vi "hmi_sistema_de_deteccion_de_fugas.vi"() -> ()   [LabVIEW 2017]
uses:
  Control 6.ctl
  <vilib>/Utility/miscctls.llb/LVBoundsTypeDef.ctl
  <vilib>/Instr/_visa.llb/VISA Configure Serial Port (Instr).vi
  <vilib>/MakerHub/LINX/LMH-LINX.lvlib
panel:
  in  "Tab Control":enum32{"HMI", "Monitorizacion de flujo"}(tab)
  out "Boolean 2":bool
  out "FUGA 1":bool
  out "FUGA 2":bool
  out "Boolean":bool
  in  "stop 2":bool
  in  "BOMBA ON/OFF":bool
  out "FT1":bool(c317)
  out "TANQUE\n FLUIDO:AGUA":dbl(slide) scale=0.0..100.0
  in  "valvula 1":bool
  in  "valvula 2":bool
  out "TEE 02":bool
  out "TUBERIA 1IN TRAMO 02":bool(c317)
  out "TEE1":bool
  out "Multi-Segment Pipe 2":T1
  out "Multi-Segment Pipe 3":bool(c317)
  out "BOMBA 1/2 HP":bool
  out "codo90":bool
  out "Multi-Segment Pipe 4":bool(c317)
  out "FT2":bool(c317)
  out "FT 1":dbl caption="L/min"
  out "FT 2":dbl caption="L/min"
  out "67.5°":bool
  out "45°":bool
  out "22.5°":bool
  out "90°":bool
  out "SENSOR FLUJO":bool
  out "67.5° 3":bool
  out "45° 3":bool
  out "22.5° 3":bool
  out "90° 3":bool
  out "SENSOR FLUJO 3":bool
  in  "Tiempo de Muestreo":string(combo)
  in  "Jump Button 4":bool
  in  "Guardar  a Excel":bool
  in  "Rango de grafica":i16(knob) scale=0.0..100.0
  out "Flujo de entrada y salida":cluster{dbl[], dbl[]}[](graph)
  out "Tiempo de Muestreo":dbl caption="s"
  in  "Jump Button 3":bool
  in  "stop":bool
  out "Freq2":dbl
  out "Freq1":dbl
  out "Cluster":T2
  in  "Puerto":refnum<visa-resource-name>="COM3"
  in  "BaudRate":i32(ring)=10 items=["9600"=9600, "19200"=19200, "38400"=38400, "57600"=57600, "74880"=74880, "115200"=115200]
  # "PVC  1\" FLUJO: AGUA"
  # "PVC  1/2\" FLUJO: AGUA"
  # "FUGA 1"
  # "2.5 m"
  # "PVC  1/2\" FLUJO: AGUA"
  # "FUGA 2"
  # "PVC  1\" FLUJO: AGUA"
  # "6 m"
  # "MONITOREO DE SENSORES DE FLUJO YF-S201"
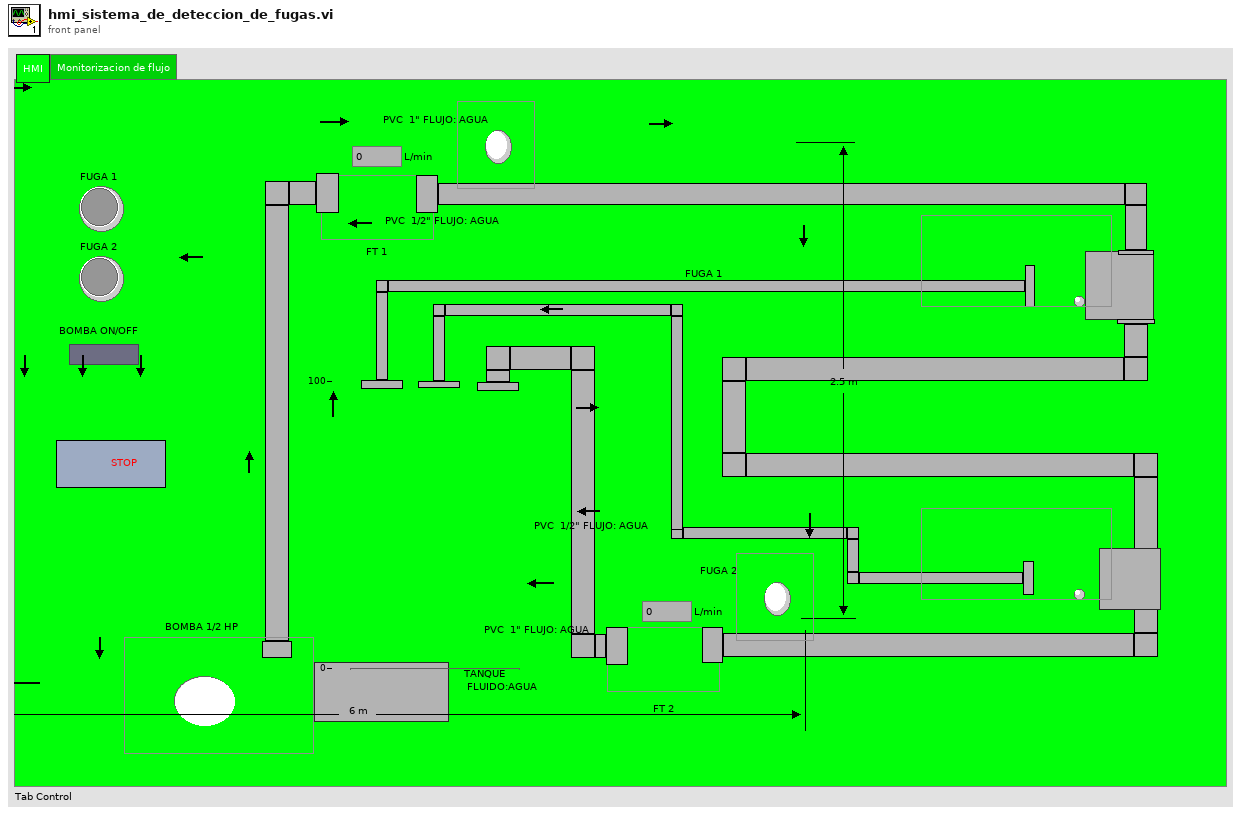
[diagram p1: front panel]
types:
  T1 = typedef "Control 6.ctl" = bool
  T2 = cluster{"FLUJO DE ENTRADA":dbl, "FLUJO DE SALIDA":dbl, "VOLUMEN 1 (L) ":dbl, "VOLUMEN 2 (L) ":dbl}
  T3 = typedef "LVBoundsTypeDef.ctl" = cluster{"Width":u32, "Height":u32}
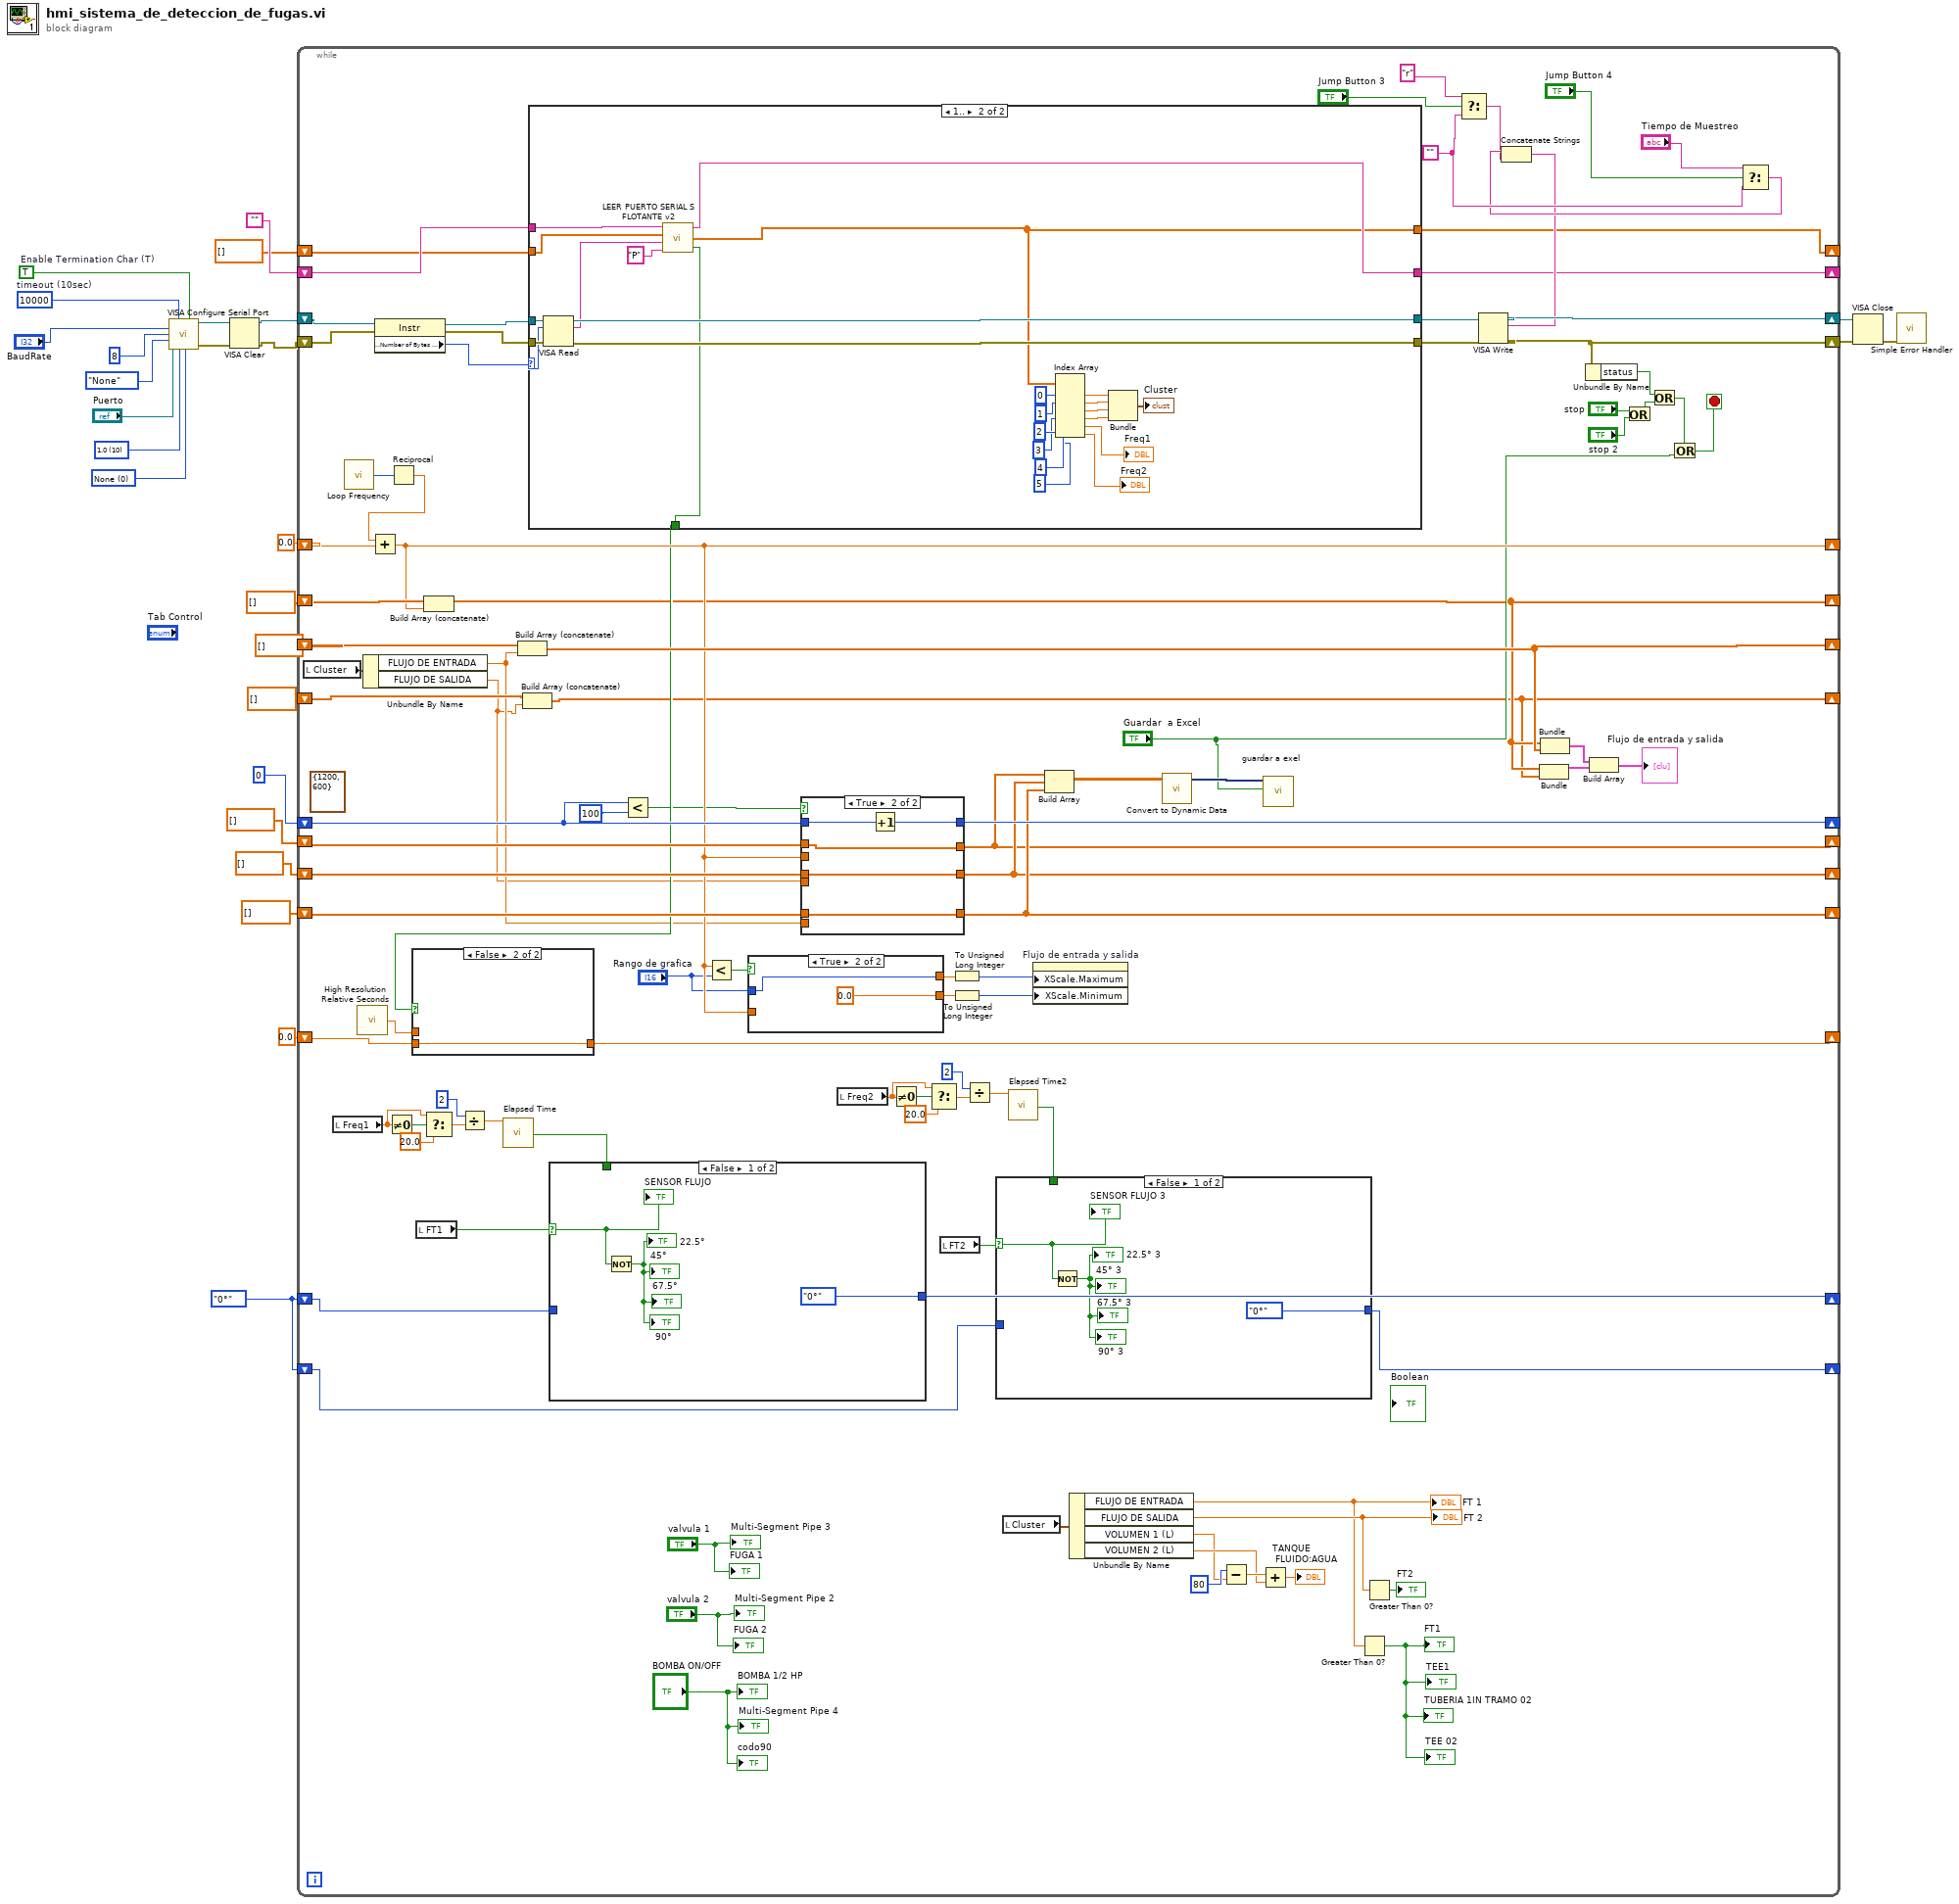
[diagram p0: block diagram]
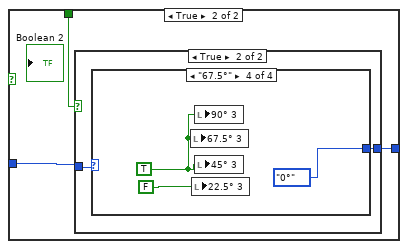
[diagram p2: hidden frame]
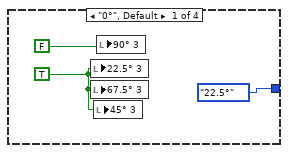
[diagram p4: hidden frame]
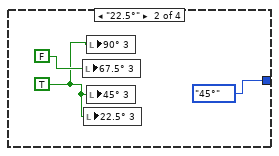
[diagram p5: hidden frame]
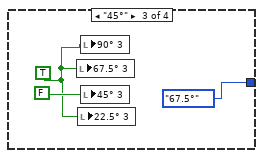
[diagram p6: hidden frame]
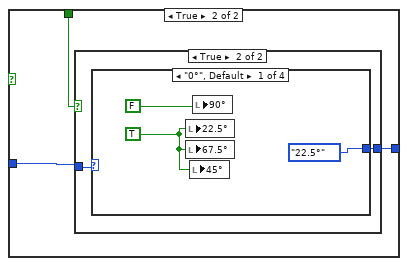
[diagram p7: hidden frame]
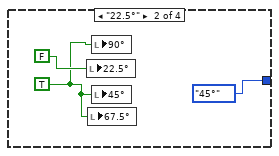
[diagram p9: hidden frame]
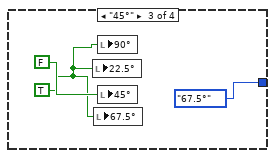
[diagram p10: hidden frame]
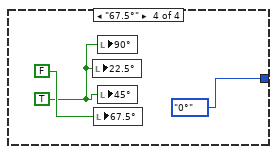
[diagram p11: hidden frame]
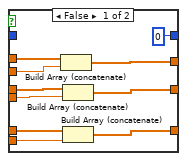
[diagram p12: hidden frame]
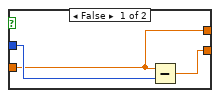
[diagram p13: hidden frame]
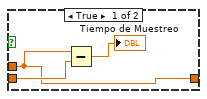
[diagram p14: hidden frame]
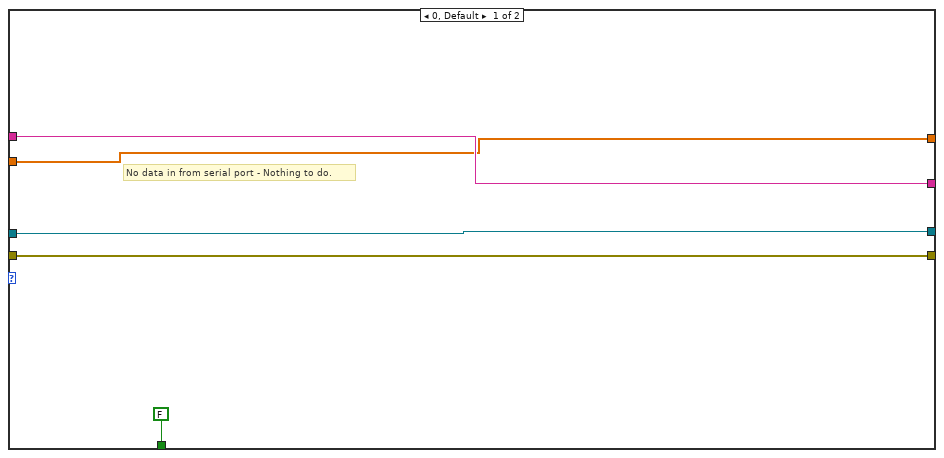
[diagram p15: hidden frame]
diagram:
  w3 = enum16{"0°", "22.5°", "45°", "67.5°"}."0°"
  w18 = u16 10 items=["1.0"=10, "1.5"=15, "2.0"=20] ("stop bits (10: 1 bit)")
  w19 = u16 0 items=["None", "XON/XOFF", "RTS/CTS", "XON/XOFF & RTS/CTS", "DTR/DSR", "XON/XOFF & DTR/DSR"] ("flow control (0:none)")
  w24 = TRUE  # Enable Termination Char (T)
  w25 = u32 10000  # timeout (10sec)
  (unwired) T3 {"Width"=1200, "Height"=600} ("Tab Control Pane Dimension")
  n1 = call-poly "VISA Configure Serial Port"("VISA resource name"="Puerto", "timeout (10sec)"=w25, "Enable Termination\nChar (T)"=w24, "baud rate (9600)"="BaudRate", "data bits (8)"=u16 8 ("Data bits (8)"), "parity (0:none)"=enum16{"None", "Odd", "Even", "Mark", "Space"}."None" ("Parity (0:none)"), "stop bits (10: 1 bit)"=w18, "flow control (0:none)"=w19) -> ("VISA resource name out"=w22:refnum<visa-resource-name>, "error out"=w23:errorcluster)  [unwired: 6 in]
  n2 = VISA Clear(VISA resource name=w22, error in (no error)=w23) -> (VISA resource name out=w21:refnum<visa-resource-name>, error out=w6:errorcluster)
  n3 = while {
    shift-right: [w72] -> _
    shift-left: dbl[] [] -> [w116]
    shift-right: [w93] -> _
    shift-left: 0.0 -> [w117]
    shift-right: [w104] -> _
    shift-left: dbl[] [] -> [w114]
    shift-right: [w71] -> _
    shift-left: dbl[] [] -> [w115]
    shift-right: [w112] -> _
    shift-left: 0.0 ("relative seconds") -> [w113]
    shift-right: [w99] -> _
    shift-left: 0 -> [w100]
    shift-right: [w94] -> _
    shift-left: dbl[] [] -> [w97]
    shift-right: [w95] -> _
    shift-left: dbl[] [] -> [w96]
    shift-right: [w92] -> _
    shift-left: dbl[] [] -> [w98]
    shift-right: [w119] -> w27
    shift-left: w6 -> [w87]
    shift-right: [w86] -> w5
    shift-left: w21 -> [w124]
    shift-right: [w57] -> _
    shift-left: w3 -> [w56]
    shift-right: [w37] -> _
    shift-left: w3 -> [w46]
    shift-right: [w30] -> _
    shift-left: "" -> [w31]
    shift-right: [w28] -> _
    shift-left: dbl[] [] -> [w29]
    stop <- w103 stop-if-true
    w85 = ""
    n4 = local read "Cluster"() -> (w70:T2)
    n5 = local read "Freq1"() -> (w54:dbl)
    n6 = call <vilib>:"Loop Frequency.vi"() -> ("Loop Rate (Hz)"=w107:u32)
    n7 = call <vilib>:"High Resolution Relative Seconds.vi"() -> ("relative seconds"=w108:dbl)
    n8 = Unbundle By Name(w70) -> ("FLUJO DE ENTRADA"=w69:dbl, "FLUJO DE SALIDA"=w68:dbl)
    n9 = property class="Instr"(reference=w124, error in=w87) -> (reference out=w126:refnum<visa-resource-name>, error out=w125:errorcluster, "Serial Settings:Number of Bytes at Serial Port"=w123:u32)
    n10 = Not Equal To 0?(x=w54) -> (x != 0?=w55:bool)
    n11 = Reciprocal(x=w107) -> (1/x=w111:dbl)
    n12 = Add(x=w111, y=w117) -> (x+y=w93:dbl)
    n13 = local read "FT1"() -> (w58:bool)
    n14 = Build Array (concatenate)(w116, w93) -> (w72:dbl[])
    n15 = Select(t=w54, s=w55, f=20.0) -> (s? t:f=w52:dbl)
    n16 = Divide(x=i8 2, y=w52) -> (x/y=w51:dbl)
    n17 = call "Elapsed Time"("Time Target (s)"=w51) -> ("Time has Elapsed"=w49:bool)  [unwired: 11 in, 7 out]
    n18 = Build Array (concatenate)(w114, w69) -> (w104:dbl[])
    n19 = Build Array (concatenate)(w115, w68) -> (w71:dbl[])
    n20 = case shown="1.." w123 {
      selector: w123 -> [_ w218]
      tunnel: [w196 w222] -> w120
      tunnel: [w197 w221] -> w121
      tunnel: w126 -> [w197 w220]
      tunnel: w125 -> [w196 w219]
      tunnel: [FALSE w203] -> w88
      tunnel: w31 -> [w194 w201]
      tunnel: [w194 w200] -> w30
      tunnel: w29 -> [w193 w199]
      tunnel: [w193 w198] -> w28
      frame 0, Default {
        # "No data in from serial port - Nothing to do."
      }
      frame 1.. {
        n21 = VISA Read(VISA resource name=w220, byte count=w218, error in (no error)=w219) -> (VISA resource name out=w221:refnum<visa-resource-name>, read buffer=w202:string, error out=w222:errorcluster)  [unwired: 1 out]
        n22 = call <userlib>:"LEER PUERTO SERIAL S FLOTANTE v2.vi"("caracter terminador"="P" ("regular expression"), "read buffer"=w202, "buffer de datos"=w199, "buffer in"=w201) -> ("indicador de llegada de datos"=w203:bool, "salida datos numericos"=w198:dbl[], "buffer out"=w200:string)
        n23 = Index Array(array=w198, index #1=0 ("index"), index #2=1 ("index"), index #3=2 ("index"), index #4=3 ("index"), index #5=4 ("index"), index #6=5 ("index")) -> (element #1=w216:dbl, element #2=w215:dbl, element #3=w213:dbl, element #4=w214:dbl, element #5=→"Freq1":dbl, element #6=→"Freq2":dbl)
        n24 = Bundle(w216, w215, w213, w214) -> (→"Cluster":cluster{dbl, dbl, dbl, dbl})  [unwired: 1 in]
      }
    }
    n25 = case shown="False" w88 {
      tunnel: w113 -> [w191 w192]
      tunnel: w108 -> [w189 _]
      tunnel: [w189 w192] -> w112
      frame True {
        n26 = Subtract(x=w189, y=w191) -> (x-y=→"Tiempo de Muestreo":dbl)
      }
      frame False {
      }
    }
    n27 = case shown="False" w58 {
      selector: w58 -> [w150 _]
      tunnel: w56 -> [_ w153]
      tunnel: [enum16{"0°", "22.5°", "45°", "67.5°"}."0°" w152] -> w57
      tunnel: w49 -> [_ w151]
      frame False {
        n28 = Not(x=w150) -> (.not. x?=→"90°" →"22.5°" →"45°" →"67.5°":bool)
        "SENSOR FLUJO" <- w150
      }
      frame True {
        n29 = case shown="True" w151 {
          tunnel: w153 -> [w154 w156]
          tunnel: [w154 w155] -> w152
          frame False {
          }
          frame True {
            n30 = case shown="\"0°\", Default" w156 {
              tunnel: [enum16{"0°", "22.5°", "45°", "67.5°"}."22.5°" enum16{"0°", "22.5°", "45°", "67.5°"}."45°" enum16{"0°", "22.5°", "45°", "67.5°"}."67.5°" enum16{"0°", "22.5°", "45°", "67.5°"}."0°"] -> w155
              frame "0°", Default {
                w157 = TRUE
                n31 = local write "22.5°"(w157) -> ()
                n32 = local write "67.5°"(w157) -> ()
                n33 = local write "45°"(w157) -> ()
                n34 = local write "90°"(FALSE) -> ()
              }
              frame "22.5°" {
                w160 = TRUE
                n35 = local write "22.5°"(FALSE) -> ()
                n36 = local write "67.5°"(w160) -> ()
                n37 = local write "90°"(w160) -> ()
                n38 = local write "45°"(w160) -> ()
              }
              frame "45°" {
                w163 = TRUE
                n39 = local write "22.5°"(w163) -> ()
                n40 = local write "67.5°"(w163) -> ()
                n41 = local write "90°"(w163) -> ()
                n42 = local write "45°"(FALSE) -> ()
              }
              frame "67.5°" {
                w166 = TRUE
                n43 = local write "22.5°"(w166) -> ()
                n44 = local write "67.5°"(FALSE) -> ()
                n45 = local write "90°"(w166) -> ()
                n46 = local write "45°"(w166) -> ()
              }
            }
          }
        }
      }
    }
    n47 = Less?(x=w100, y=u32 100) -> (x < y?=w73:bool)
    n48 = Less?(x=w93, y="Rango de grafica") -> (x < y?=w106:bool)
    n49 = case shown="True" w106 {
      tunnel: "Rango de grafica" -> [w185 w187]
      tunnel: [w184 w187] -> w78
      tunnel: [w186 0.0] -> w76
      tunnel: w93 -> [w184 _]
      frame False {
        n50 = Subtract(x=w184, y=w185) -> (x-y=w186:dbl)
      }
      frame True {
      }
    }
    n51 = case shown="True" w73 {
      tunnel: w100 -> [_ w183]
      tunnel: [u32 0 w182] -> w99
      tunnel: w98 -> [w177 w179]
      tunnel: w68 -> [w175 _]
      tunnel: [w178 w181] -> w94
      tunnel: w97 -> [w176 w181]
      tunnel: w69 -> [w173 _]
      tunnel: w96 -> [w174 w180]
      tunnel: [w172 w180] -> w95
      tunnel: [w171 w179] -> w92
      tunnel: w93 -> [w170 _]
      frame False {
        n52 = Build Array (concatenate)(w177, w170) -> (w171:dbl[])
        n53 = Build Array (concatenate)(w176, w175) -> (w178:dbl[])
        n54 = Build Array (concatenate)(w174, w173) -> (w172:dbl[])
      }
      frame True {
        n55 = Increment(x=w183) -> (x+1=w182:u32)
      }
    }
    n56 = local read "Freq2"() -> (w44:dbl)
    n57 = Not Equal To 0?(x=w44) -> (x != 0?=w45:bool)
    n58 = Select(t=w44, s=w45, f=20.0) -> (s? t:f=w42:dbl)
    n59 = local read "FT2"() -> (w38:bool)
    n60 = To Unsigned Long Integer(number=w78) -> (unsigned 32bit integer=w77:u32)
    n61 = To Unsigned Long Integer(number=w76) -> (unsigned 32bit integer=w75:u32)
    n62 = Divide(x=i8 2, y=w42) -> (x/y=w41:dbl)
    n63 = local read "Cluster"() -> (w60:T2)
    n64 = call "Elapsed Time2"("Time Target (s)"=w41) -> ("Time has Elapsed"=w39:bool)  [unwired: 11 in, 7 out]
    n65 = case shown="False" w38 {
      selector: w38 -> [w129 _]
      tunnel: w46 -> [_ w132]
      tunnel: [enum16{"0°", "22.5°", "45°", "67.5°"}."0°" w131] -> w37
      tunnel: w39 -> [_ w130]
      frame False {
        n66 = Not(x=w129) -> (.not. x?=→"90° 3" →"22.5° 3" →"45° 3" →"67.5° 3":bool)
        "SENSOR FLUJO 3" <- w129
      }
      frame True {
        n67 = case shown="True" w130 {
          tunnel: w132 -> [w133 w135]
          tunnel: [w133 w134] -> w131
          frame False {
          }
          frame True {
            n68 = case shown="\"67.5°\"" w135 {
              tunnel: [enum16{"0°", "22.5°", "45°", "67.5°"}."22.5°" enum16{"0°", "22.5°", "45°", "67.5°"}."45°" enum16{"0°", "22.5°", "45°", "67.5°"}."67.5°" enum16{"0°", "22.5°", "45°", "67.5°"}."0°"] -> w134
              frame "0°", Default {
                w136 = TRUE
                n69 = local write "22.5° 3"(w136) -> ()
                n70 = local write "67.5° 3"(w136) -> ()
                n71 = local write "45° 3"(w136) -> ()
                n72 = local write "90° 3"(FALSE) -> ()
              }
              frame "22.5°" {
                w139 = TRUE
                n73 = local write "67.5° 3"(FALSE) -> ()
                n74 = local write "22.5° 3"(w139) -> ()
                n75 = local write "90° 3"(w139) -> ()
                n76 = local write "45° 3"(w139) -> ()
              }
              frame "45°" {
                w142 = TRUE
                n77 = local write "67.5° 3"(w142) -> ()
                n78 = local write "22.5° 3"(w142) -> ()
                n79 = local write "90° 3"(w142) -> ()
                n80 = local write "45° 3"(FALSE) -> ()
              }
              frame "67.5°" {
                w145 = TRUE
                n81 = local write "67.5° 3"(w145) -> ()
                n82 = local write "22.5° 3"(FALSE) -> ()
                n83 = local write "90° 3"(w145) -> ()
                n84 = local write "45° 3"(w145) -> ()
              }
            }
          }
        }
      }
    }
    n85 = property on="Flujo de entrada y salida" class="XYGraph (strict)"("XScale.Maximum"=w77, "XScale.Minimum"=w75) -> ()  [unwired: 2 in, 2 out]
    n86 = Build Array(w92, w94, w95) -> (w90:dbl[][])
    n87 = Unbundle By Name(w60) -> ("FLUJO DE ENTRADA"=w59:dbl, "FLUJO DE SALIDA"=w66:dbl, "VOLUMEN 1 (L)"=w35:dbl, "VOLUMEN 2 (L)"=w61:dbl)
    "FT 1" <- w59
    "FT 2" <- w66
    n88 = call "Convert to Dynamic Data"("2D Array"=w90) -> ("Dynamic Data Type"=w91:dynamicdata)  [unwired: 3 in]
    n89 = Subtract(x=80, y=w35) -> (x-y=w62:dbl)
    n90 = Add(x=w62, y=w61) -> (x+y=→"TANQUE\n FLUIDO:AGUA":dbl)
    n91 = call "guardar a exel"("Signals"=w91, "Enable"="Guardar  a Excel") -> ()  [unwired: 15 in, 3 out]
    n92 = Greater Than 0?(x=w59) -> (x > 0?=→"TUBERIA 1IN TRAMO 02" →"TEE1" →"TEE 02" →"FT1":bool)
    n93 = Greater Than 0?(x=w66) -> (x > 0?=→"FT2":bool)
    n94 = Select(t="r", s="Jump Button 3", f=w85) -> (s? t:f=w82:string)
    n95 = Bundle(w72, w71) -> (w109:cluster{dbl[], dbl[]})  [unwired: 1 in]
    n96 = Bundle(w72, w104) -> (w110:cluster{dbl[], dbl[]})  [unwired: 1 in]
    n97 = Build Array(w110, w109) -> (→"Flujo de entrada y salida":cluster{dbl[], dbl[]}[])
    n98 = Or(x="stop", y="stop 2") -> (x .or. y?=w34:bool)
    n99 = Select(t="Tiempo de Muestreo", s="Jump Button 4", f=w85) -> (s? t:f=w83:string)
    n100 = Concatenate Strings(w83, w82) -> (w80:string)
    n101 = VISA Write(VISA resource name=w121, write buffer=w80, error in (no error)=w120) -> (VISA resource name out=w86:refnum<visa-resource-name>, error out=w119:errorcluster)  [unwired: 1 out]
    n102 = Unbundle By Name(w119) -> ("status"=w122:bool)
    n103 = Or(x=w122, y=w34) -> (x .or. y?=w102:bool)
    n104 = Or(x=w102, y="Guardar  a Excel") -> (x .or. y?=w103:bool)
    "BOMBA 1/2 HP" <- "BOMBA ON/OFF"
    "codo90" <- "BOMBA ON/OFF"
    "Multi-Segment Pipe 4" <- "BOMBA ON/OFF"
    "Multi-Segment Pipe 3" <- "valvula 1"
    "Multi-Segment Pipe 2" <- "valvula 2"
    "FUGA 2" <- "valvula 2"
    "FUGA 1" <- "valvula 1"
  }
  n105 = VISA Close(VISA resource name=w5, error in (no error)=w27) -> (error out=w26:errorcluster)
  n106 = call <vilib>:"Simple Error Handler.vi"("error in (no error)"=w26) -> ()  [unwired: 4 in, 5 out]
